vi "CAL-Read Data.vi"(0 "user path":path, 11 "error in (no error)":errorcluster) -> (4 "Frequency (Hz)":dbl[](array[numeric]), 6 "Mag":dbl[](array[numeric]), 8 "Phase":dbl[](array[numeric]), 14 "Fs (Hz)":dbl, 15 "error out":errorcluster)   [LabVIEW 2020]
uses:
  <vilib>/regexp/Match Regular Expression.xnode
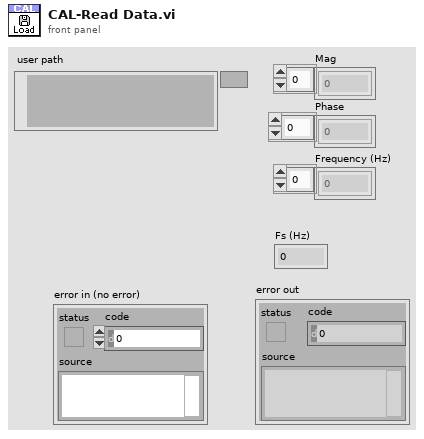
[diagram p1: front panel]
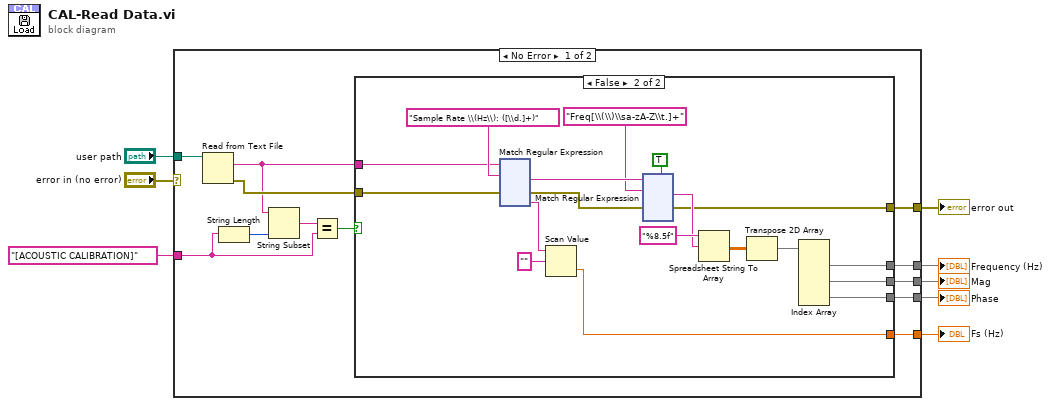
[diagram p0: block diagram]
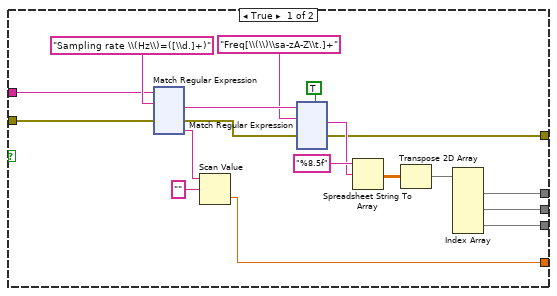
[diagram p2: hidden frame]
diagram:
  n1 = case shown="No Error" "error in (no error)" {
    selector: "error in (no error)" -> [_ w521]
    tunnel: "user path" -> [w20 _]
    tunnel: [w14 w521] -> w6
    tunnel: [w19 _] -> w5
    tunnel: [w18 _] -> w4
    tunnel: [w17 _] -> w3
    tunnel: [w15 _] -> w2
    tunnel: "[ACOUSTIC CALIBRATION]" -> [w10 _]
    frame No Error {
      n2 = Read from Text File(file (use dialog)=w20) -> (text=w13:string, error out=w16:errorcluster)  [unwired: 3 in, 2 out]
      n3 = String Length(string=w10) -> (length=w12:i32)
      n4 = String Subset(string=w13, length (rest)=w12) -> (substring=w11:string)  [unwired: 1 in]
      n5 = Equal?(x=w11, y=w10) -> (x = y?=w9:bool)
      n6 = case shown="False" w9 {
        tunnel: [w38 w288] -> w19
        tunnel: [w37 w287] -> w18
        tunnel: [w36 w286] -> w17
        tunnel: w16 -> [w32 w282]
        tunnel: [w28 w278] -> w15
        tunnel: [w23 w273] -> w14
        tunnel: w13 -> [w21 w271]
        frame True {
          n7 = xnode "Match Regular Expression"("input string"=w21, "regular expression"="Sampling rate \\(Hz\\)=([\\d.]+)", "error in"=w32) -> ("after match"=w27:string, "error out"=w24:errorcluster, "submatch 1"=w30:string)  [unwired: 3 in, 3 out]
          n8 = Scan Value(string=w30, format string="") -> (value=w28:dbl)  [unwired: 1 in, 1 out]
          n9 = xnode "Match Regular Expression"("input string"=w27, "regular expression"="Freq[\\(\\)\\sa-zA-Z\\t.]+", "error in"=w24, "multiline? (F)"=TRUE) -> ("after match"=w25:string, "error out"=w23:errorcluster)  [unwired: 2 in, 4 out]
          n10 = Spreadsheet String To Array(format string="%8.5f" ("format (%.3f)"), spreadsheet string=w25) -> (array=w34:dbl[][])  [unwired: 2 in]
          n11 = Transpose 2D Array(2D array=w34) -> (transposed array=w33:dbl[][])
          n12 = Index Array(array=w33) -> (element #1=w38:dbl[], element #2=w37:dbl[], element #3=w36:dbl[])  [unwired: 6 in]
        }
        frame False {
          n13 = xnode "Match Regular Expression"("input string"=w271, "regular expression"="Sample Rate \\(Hz\\): ([\\d.]+)", "error in"=w282) -> ("after match"=w277:string, "error out"=w274:errorcluster, "submatch 1"=w280:string)  [unwired: 3 in, 3 out]
          n14 = Scan Value(string=w280, format string="") -> (value=w278:dbl)  [unwired: 1 in, 1 out]
          n15 = xnode "Match Regular Expression"("input string"=w277, "regular expression"="Freq[\\(\\)\\sa-zA-Z\\t.]+", "error in"=w274, "multiline? (F)"=TRUE) -> ("after match"=w275:string, "error out"=w273:errorcluster)  [unwired: 2 in, 4 out]
          n16 = Spreadsheet String To Array(format string="%8.5f" ("format (%.3f)"), spreadsheet string=w275) -> (array=w284:dbl[][])  [unwired: 2 in]
          n17 = Transpose 2D Array(2D array=w284) -> (transposed array=w283:dbl[][])
          n18 = Index Array(array=w283) -> (element #1=w288:dbl[], element #2=w287:dbl[], element #3=w286:dbl[])  [unwired: 6 in]
        }
      }
    }
    frame Error {
    }
  }
  "error out" <- w6
  "Frequency (Hz)" <- w5
  "Mag" <- w4
  "Phase" <- w3
  "Fs (Hz)" <- w2
